vi "Amplitude and Levels N chan (obs).vi"(6 "state settings":T1={"method"=enum."auto select", "histogram size"=256, "histogram method"=enum."mode", "reserved"=1.0} {"reserved" format="%0.2f"}, 8 "error in (no error)":errorcluster, 11 "signal(s) in":waveform(dbl)[](array[waveform])) -> (0 "error out":errorcluster, 1 "low state level":dbl[](array[numeric]) format="%.2p", 2 "high state level":dbl[](array[numeric]) format="%.2p", 3 "amplitude":dbl[](array[numeric]) format="%.2p")   [LabVIEW 2020, in "NI_MAPro.lvlib"]
uses:
  NI_MAPro.lvlib
  NI_MABase.lvlib
panel:
  # "This VI is obsolete !!!\nYou should replace this VI in your diagram with the Amplitude and Levels VI."
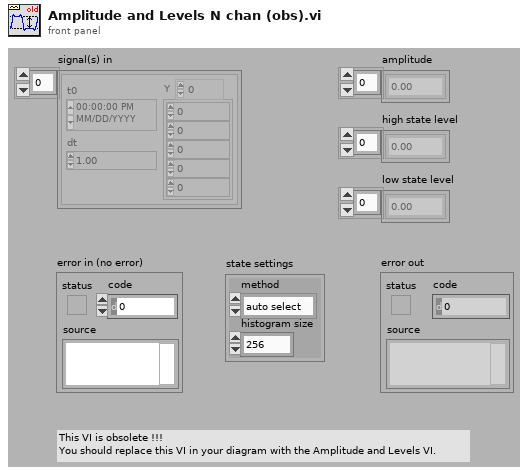
[diagram p1: front panel]
types:
  T1 = cluster{"method":enum32{"histogram", "peak", "auto select"}, "histogram size":i32, "histogram method":enum16{"mode"}, "reserved":dbl}
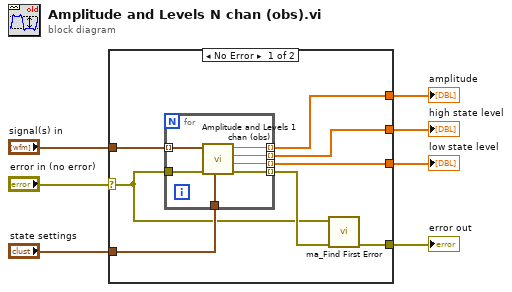
[diagram p0: block diagram]
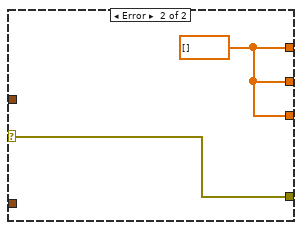
[diagram p2: hidden frame]
diagram:
  n1 = case shown="No Error" "error in (no error)" {
    selector: "error in (no error)" -> [w9 w24]
    tunnel: "state settings" -> [w14 _]
    tunnel: [w8 w24] -> w5
    tunnel: "signal(s) in" -> [w15 _]
    tunnel: [w13 w23] -> w3
    tunnel: [w12 w23] -> w2
    tunnel: [w11 w23] -> w1
    frame No Error {
      n2 = for {
        tunnel: w9 -> [w20]
        tunnel: w14 -> [w22]
        tunnel: [w16] -> w10 mode=indexing
        tunnel: [w19] -> w13 mode=indexing
        tunnel: [w18] -> w12 mode=indexing
        tunnel: [w17] -> w11 mode=indexing
        tunnel: w15 -> [w21] mode=indexing
        n3 = call "Amplitude and Levels 1 chan (obs).vi"("state settings"=w22, "error in (no error)"=w20, "signal in"=w21) -> ("error out"=w16:errorcluster, "low state level"=w17:dbl, "high state level"=w18:dbl, "amplitude"=w19:dbl)  [unwired: 5 out]
      }
      n4 = call "ma_Find First Error.vi"("error array in"=w10, "error in 1 (no error)"=w9) -> ("error out"=w8:errorcluster)  [unwired: 2 in, 3 out]
    }
    frame Error {
      w23 = dbl[] []
    }
  }
  "error out" <- w5
  "amplitude" <- w3
  "high state level" <- w2
  "low state level" <- w1
